vi "Sim_Config.vi"(7 "Hardware Case Selection":enum16{"Init", "Read", "Write", "Close"}(ring), 8 "error in (no error)":errorcluster, 11 "?":T1={"Session_array"=[{"Add Bearer"=FALSE, "APN Name\n"="", "AMBR Uplink(Gbps)\n"="", "AMBR Downlink(Gbps)\n"="", "Session name"="", "Bearer_Array"=[], "Delete Session"=FALSE}], "SIM_U_Config"={"Add"=FALSE, "Close"=FALSE, "SIM_UI"=[], "Save"=FALSE}}) -> (0 "error out":errorcluster, 3 "Cluster":T1)   [LabVIEW 2021]
uses:
  Sim_Confi.ctl
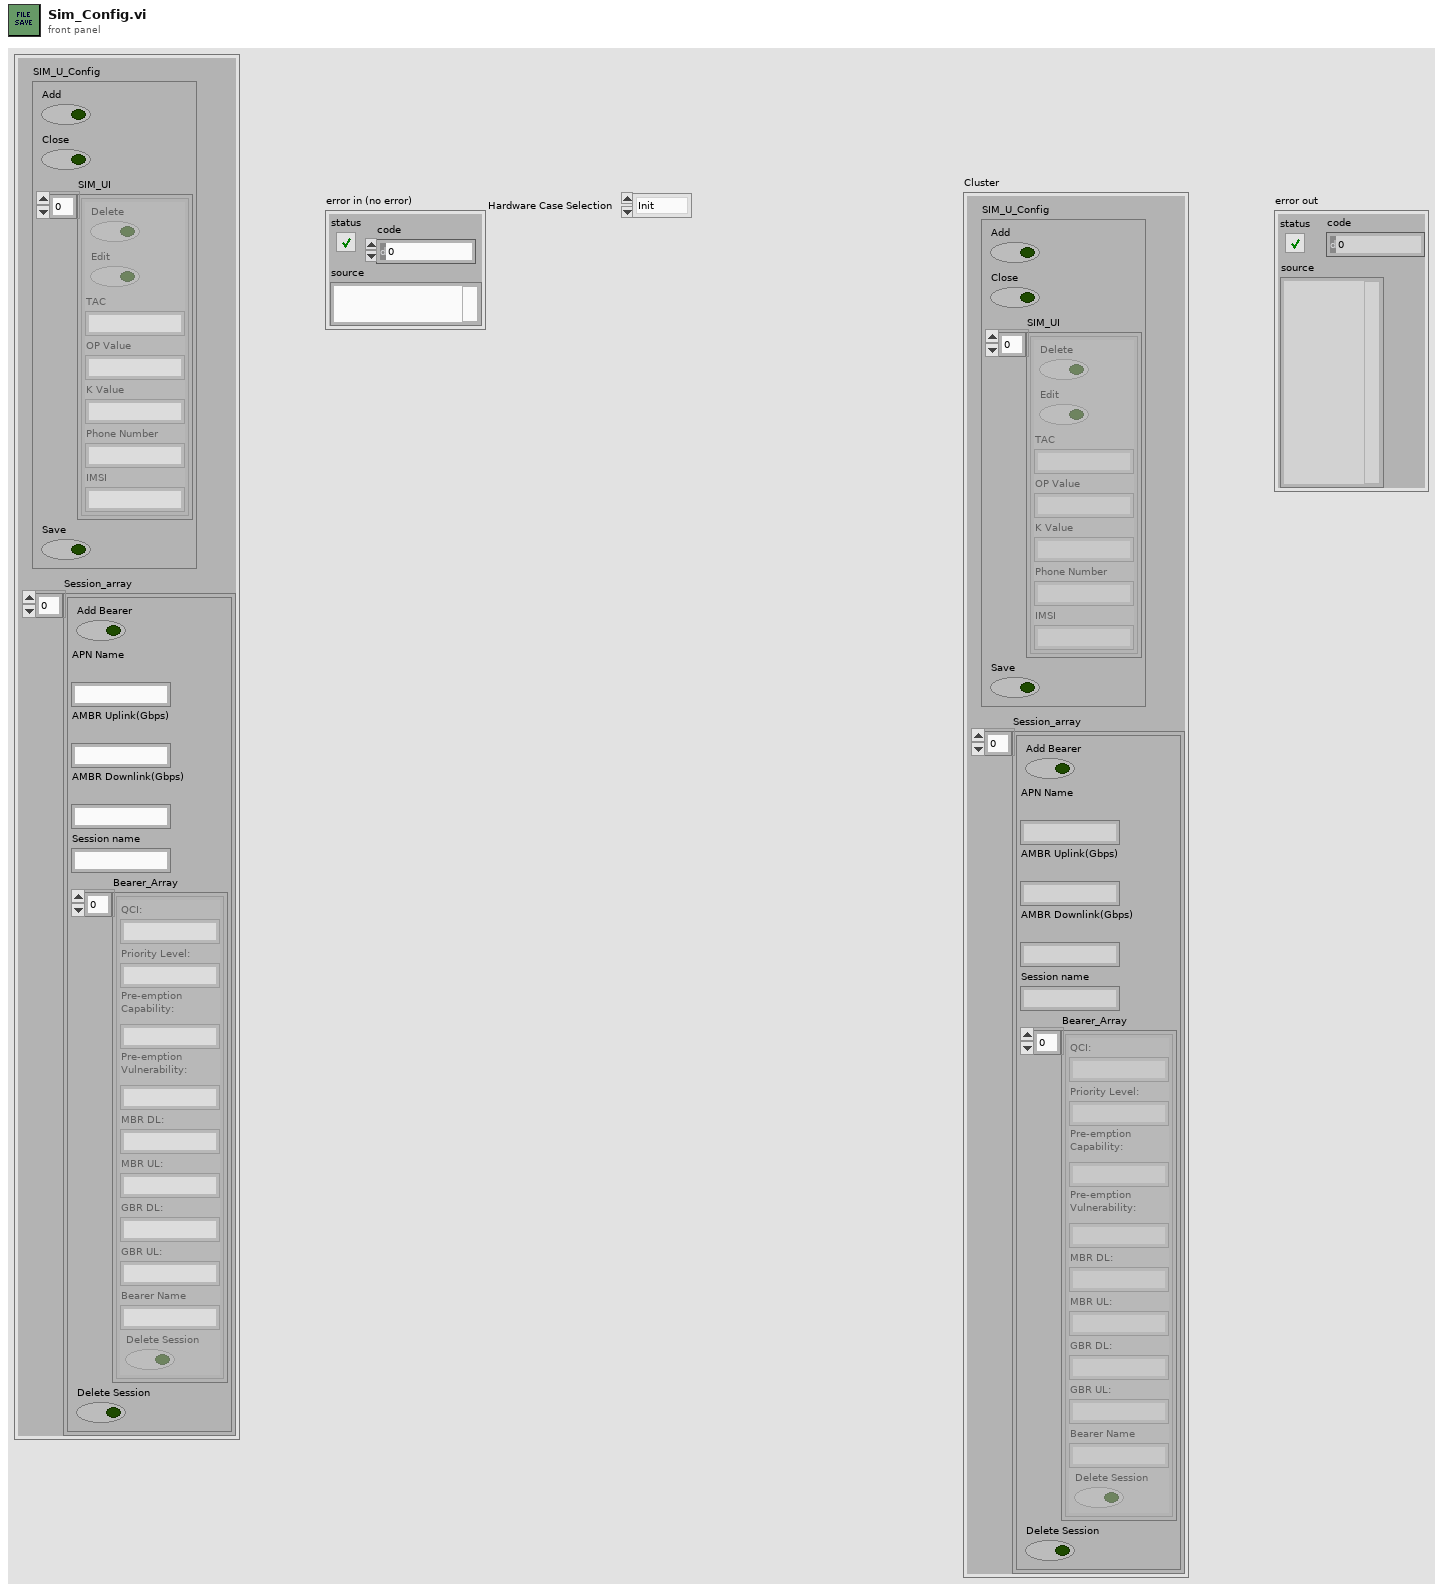
[diagram p1: front panel]
types:
  T1 = typedef "Sim_Confi.ctl" = cluster{"Session_array":cluster{"Add Bearer":bool, "APN Name\n":string, "AMBR Uplink(Gbps)\n":string, "AMBR Downlink(Gbps)\n":string, "Session name":string, "Bearer_Array":cluster{"QCI:":string, "Priority Level:":string, "Pre-emption\nCapability:":string, "Pre-emption\nVulnerability:":string, "MBR DL:":string, "MBR UL:":string, "GBR DL:":string, "GBR UL:":string, "Bearer Name":string, "Delete Session":bool}[], "Delete Session":bool}[], "SIM_U_Config":cluster{"Add":bool, "Close":bool, "SIM_UI":cluster{"Delete":bool, "Edit":bool, "TAC":string, "OP Value":string, "K Value":string, "Phone Number":string, "IMSI":string}[], "Save":bool}}
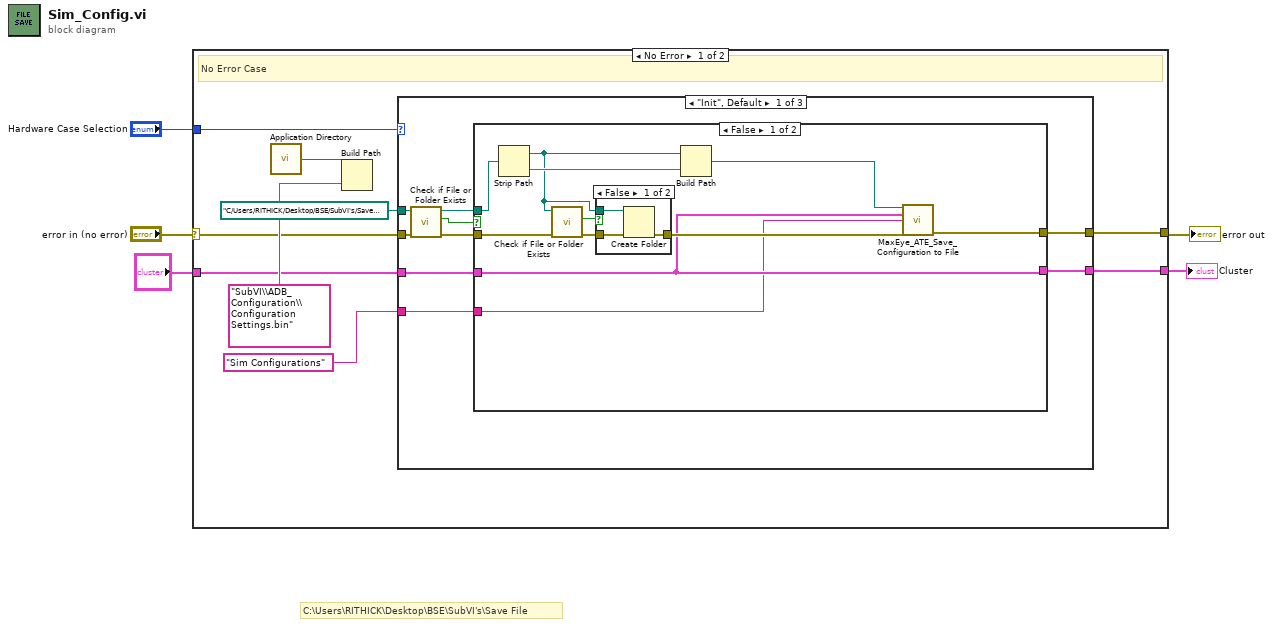
[diagram p0: block diagram]
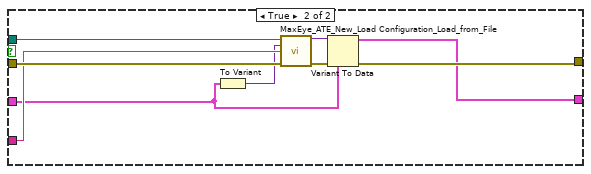
[diagram p3: hidden frame]
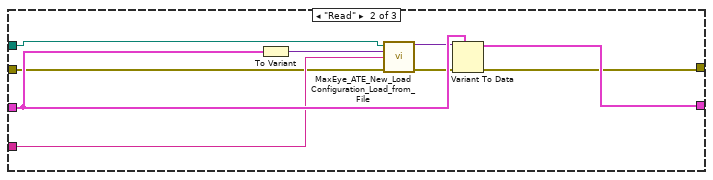
[diagram p4: hidden frame]
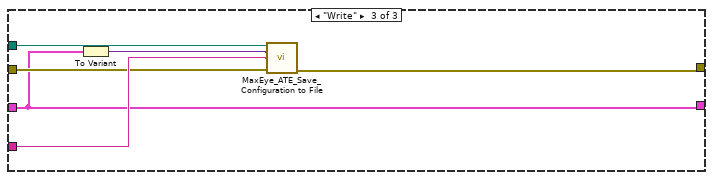
[diagram p5: hidden frame]
diagram:
  # "C:\\Users\\RITHICK\\Desktop\\BSE\\SubVI's\\Save File"
  n1 = case shown="No Error" "error in (no error)" {
    selector: "error in (no error)" -> [w12 w64]
    tunnel: [w11 w64] -> w5
    tunnel: [w10 w63] -> w1
    tunnel: "Hardware Case Selection" -> [w9 _]
    tunnel: "?" -> [w8 w63]
    frame No Error {
      # "No Error Case"
      n2 = call <vilib>:"Application Directory.vi"() -> ("Application Directory"=w14:path)
      n3 = Build Path(base path=w14, name or relative path="SubVI\\ADB_Configuration\\Configuration Settings.bin") -> ()  [unwired: 1 out]
      n4 = case shown="\"Init\", Default" w9 {
        tunnel: path "C:/Users/RITHICK/Desktop/BSE/SubVI's/Save File/Sim Configurations/Sim Configurations.bin" ("appended path") -> [w23 w53 w62]
        tunnel: w12 -> [w22 w48 w59]
        tunnel: [w20 w54 w58] -> w11
        tunnel: [w19 w55 w57] -> w10
        tunnel: w8 -> [w17 w56 w57]
        tunnel: "Sim Configurations" ("Config Header") -> [w16 w51 w60]
        frame "Init", Default {
          n5 = call <vilib>:"Check if File or Folder Exists.vi"("error in (no error)"=w22, "path"=w23) -> ("error out"=w21:errorcluster, "file or folder exists?"=w18:bool, "dup path"=w15:path)  [unwired: 7 in]
          n6 = case shown="False" w18 {
            tunnel: w21 -> [w33 w43]
            tunnel: w15 -> [w24 w41]
            tunnel: [w28 w47] -> w20
            tunnel: [w26 w46] -> w19
            tunnel: w17 -> [w26 w39]
            tunnel: w16 -> [w25 w42]
            frame False {
              n7 = Strip Path(path=w24) -> (stripped path=w30:path, name=w34:string)
              n8 = call <vilib>:"Check if File or Folder Exists.vi"("error in (no error)"=w33, "path"=w30) -> ("error out"=w32:errorcluster, "file or folder exists?"=w31:bool)  [unwired: 7 in, 1 out]
              n9 = case shown="False" w31 {
                tunnel: w32 -> [w37 w38]
                tunnel: w30 -> [w36 _]
                tunnel: [w35 w38] -> w29
                frame False {
                  n10 = Create Folder(path (use dialog)=w36, error in=w37) -> (error out=w35:errorcluster)  [unwired: 1 in, 2 out]
                }
                frame True {
                }
              }
              n11 = Build Path(base path=w30, name or relative path=w34) -> (appended path=w27:path)
              n12 = call "MaxEye_ATE_Save_Configuration to File.vi"("file path (use dialog)"=w27, "Variant"=w26, "Config Header"=w25, "error in (no error)"=w29) -> ("error out"=w28:errorcluster)  [unwired: 11 in]
            }
            frame True {
              n13 = To Variant(anything=w39) -> (Variant=w40:variant)
              n14 = call "MaxEye_ATE_New_Load Configuration_Load_from_File.vi"("file path (use dialog)"=w41, "Variant In"=w40, "Config Header"=w42, "error in (no error)"=w43) -> ("Variant Out"=w45:variant, "error out"=w44:errorcluster)  [unwired: 10 in]
              n15 = Variant To Data(error in=w44, type=w39, Variant=w45) -> (data=w46:T1, error out=w47:errorcluster)
            }
          }
        }
        frame "Read" {
          n16 = To Variant(anything=w56) -> (Variant=w52:variant)
          n17 = call "MaxEye_ATE_New_Load Configuration_Load_from_File.vi"("file path (use dialog)"=w53, "Variant In"=w52, "Config Header"=w51, "error in (no error)"=w48) -> ("Variant Out"=w50:variant, "error out"=w49:errorcluster)  [unwired: 10 in]
          n18 = Variant To Data(error in=w49, type=w56, Variant=w50) -> (data=w55:T1, error out=w54:errorcluster)
        }
        frame "Write" {
          n19 = To Variant(anything=w57) -> (Variant=w61:variant)
          n20 = call "MaxEye_ATE_Save_Configuration to File.vi"("file path (use dialog)"=w62, "Variant"=w61, "Config Header"=w60, "error in (no error)"=w59) -> ("error out"=w58:errorcluster)  [unwired: 11 in]
        }
      }
    }
    frame Error {
      # "Error case"
    }
  }
  "error out" <- w5
  "Cluster" <- w1
